vi "QuerySensors.vi"(0 "Subnet in":refnum<class "Subnet.lvclass">) -> (4 "Subnet out":refnum<class "Subnet.lvclass">, 6 "BroadcastCounter":u8, 8 "ValidCRC":i32, 10 "InvalidCRC":i32, 13 "CRCIssues":T1[](array[typedef]) {"Data" format="%02x"}, 14 "Messages":i32, 15 "error out":errorcluster)   [LabVIEW 2016]
uses:
  Subnet/Subnet.lvclass
  Common_RT_Modbus/DataTypes/RxFrame.ctl
  Subnet/Subnet.lvclass/Subnet.ctl
  Common_RT_Modbus/RTModbus.lvlib
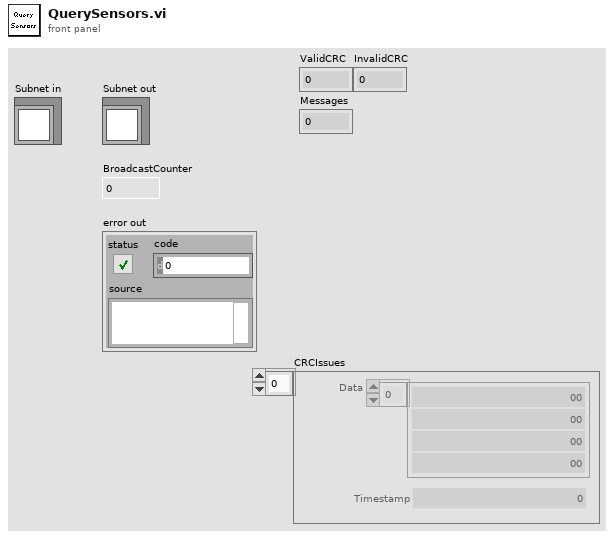
[diagram p1: front panel]
types:
  T1 = typedef "RTModbus.lvlib/RxFrame.ctl" = cluster{"Data":u8[], "Timestamp":u64}
  T2 = typedef "SubnetData.ctl" = cluster{"SubnetConstants":T3, "SubnetCommand":T6, "SubnetTelemetry":T7}
  T3 = typedef "SubnetConstants.ctl" = cluster{"Modbus":refnum<class "IModbus.lvclass">, "HPs":refnum<class "HPILC.lvclass">[], "AddressToActuator":T4[], "MTs":refnum<class "MTILC.lvclass">[], "MDs":refnum<class "MDILC.lvclass">[], "MIs":refnum<class "MIILC.lvclass">[]}
  T4 = typedef "ILCIndexData.ctl" = cluster{"ILCTypes":T5, "Index":i32}
  T5 = typedef "ILCTypes.ctl" = enum16{"Undefined", "SAA", "DAA", "HP", "MT", "MD", "MI"}
  T6 = typedef "SubnetCommand.ctl" = cluster{"BroadcastCounter":u8}
  T7 = typedef "SubnetTelemetry.ctl" = cluster{"BytesTransmitted":u32, "FramesTransmitted":u32, "BytesReceived":u32, "FramesReceived":u32, "TxInternalFIFOOverflow":bool, "InvalidInstruction":bool, "WaitForRxFrameTimeout":bool, "StartBitError":bool, "StopBitError":bool, "RxDataFIFOOverflow":bool}
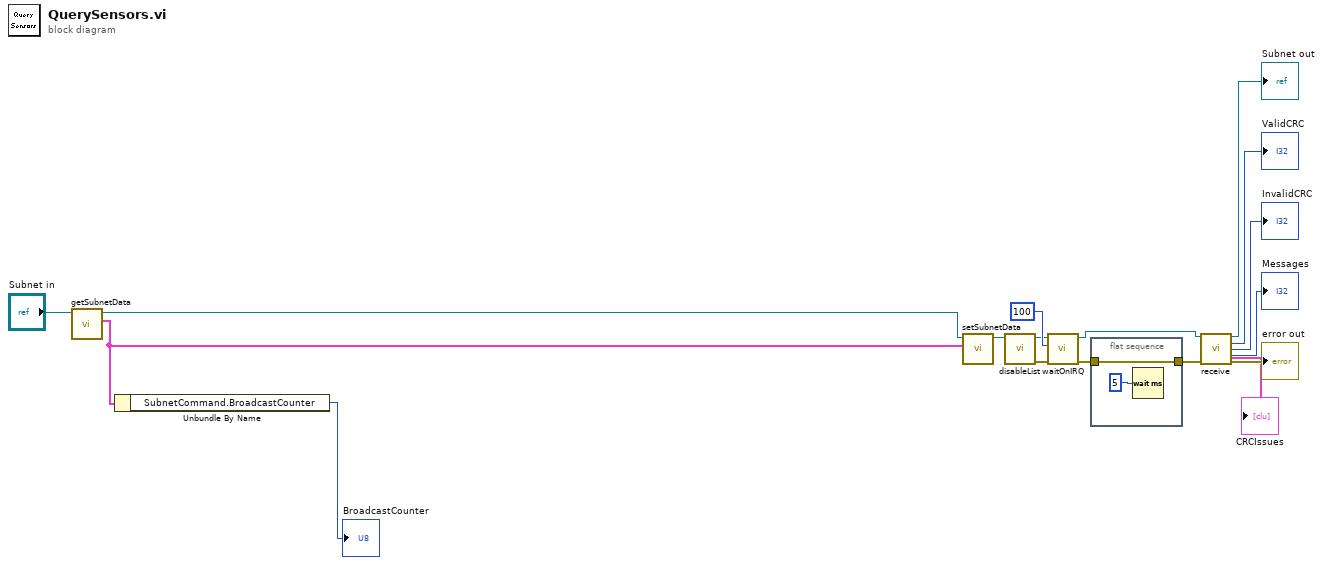
[diagram p0: block diagram]
diagram:
  n1 = call "getSubnetData.vi"("Subnet in"="Subnet in") -> ("SubnetData"=w9:T2, "Subnet out"=w10:refnum<class "Subnet.lvclass">)  [unwired: 9 in]
  n2 = Unbundle By Name(w9) -> ("SubnetCommand.BroadcastCounter"=→"BroadcastCounter":u8)
  n3 = call "setSubnetData.vi"("SubnetData"=w9, "Subnet in"=w10) -> ("Subnet out"=w11:refnum<class "Subnet.lvclass">)  [unwired: 9 in]
  n4 = call-dynamic "disableList.vi"("Subnet in"=w11) -> ("error out"=w12:errorcluster, "Subnet out"=w7:refnum<class "Subnet.lvclass">)  [unwired: 9 in]
  n5 = call-dynamic "waitOnIRQ.vi"("error in (no error)"=w12, "Timeout (ms)"=100, "Subnet in"=w7) -> ("error out"=w3:errorcluster, "Subnet out"=w13:refnum<class "Subnet.lvclass">)  [unwired: 7 in]
  n6 = flat-sequence {
    tunnel: w3 -> [w18]
    tunnel: [w18] -> w2
    frame #0 {
      n7 = Wait (ms)(milliseconds to wait=u32 5) -> ()  [unwired: 1 out]
    }
  }
  n8 = call-dynamic "receive.vi"("Subnet in"=w13, "error in (no error)"=w2) -> ("Subnet out"=→"Subnet out":refnum<class "Subnet.lvclass">, "ValidCRC"=→"ValidCRC":i32, "InvalidCRC"=→"InvalidCRC":i32, "Messages"=→"Messages":i32, "CRCIssues"=→"CRCIssues":T1[], "error out"=→"error out":errorcluster)  [unwired: 8 in]
